vi "OPC UA Server.vi"() -> ()   [LabVIEW 2018]
uses:
  <vilib>/OPCUA/controls/Data Type.ctl
  <vilib>/OPCUA/NI OPC UA Server.lvlib
panel:
  in  "stop":bool
  out "Item Path":string
  out "Server Endpoint URL":string
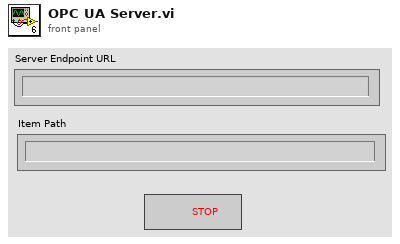
[diagram p1: front panel]
types:
  T1 = typedef "Data Type.ctl" = u16
  T2 = cluster{"name":string, "data type":T1, "access level":u16, "description":string}
  T3 = typedef "OPC UA Server Refnum.ctl" = refnum<k21>
  T4 = typedef "NodeId.ctl" = string
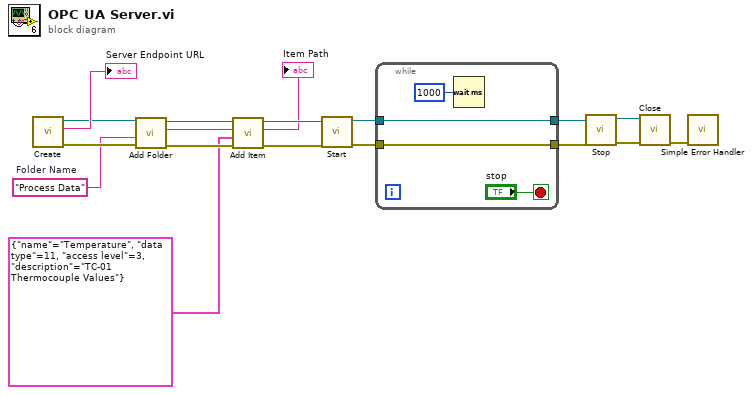
[diagram p0: block diagram]
diagram:
  w11 = "Process Data"  # Folder Name
  n1 = call <vilib>:"Create.vi"() -> ("error out"=w17:errorcluster, "server endpoint URL"=→"Server Endpoint URL":string, "OPC UA server refnum out"=w15:T3)  [unwired: 9 in]
  n2 = call <vilib>:"Add Folder.vi"("error in (no error)"=w17, "folder name"=w11, "OPC UA server refnum in"=w15) -> ("error out"=w16:errorcluster, "folder node ID"=w1:T4, "OPC UA server refnum out"=w14:T3)  [unwired: 5 in]
  n3 = call <vilib>:"Add Item.vi"("error in (no error)"=w16, "item"=T2 {"name"="Temperature", "data type"=11, "access level"=3, "description"="TC-01 Thermocouple Values"}, "parent folder node ID"=w1, "OPC UA server refnum in"=w14) -> ("error out"=w12:errorcluster, "item node ID"=→"Item Path":T4, "OPC UA server refnum out"=w13:T3)  [unwired: 3 in, 1 out]
  n4 = call <vilib>:"Start.vi"("error in (no error)"=w12, "OPC UA server refnum in"=w13) -> ("error out"=w8:errorcluster, "OPC UA server refnum out"=w6:T3)  [unwired: 7 in, 1 out]
  n5 = while {
    tunnel: w8 -> [w20]
    tunnel: [w20] -> w7
    tunnel: [w19] -> w5
    tunnel: w6 -> [w19]
    stop <- "stop" stop-if-true
    n6 = Wait (ms)(milliseconds to wait=u32 1000) -> ()  [unwired: 1 out]
  }
  n7 = call <vilib>:"Stop.vi"("error in (no error)"=w7, "OPC UA server refnum in"=w5) -> ("error out"=w4:errorcluster, "OPC UA server refnum out"=w3:T3)  [unwired: 8 in]
  n8 = call <vilib>:"Close.vi"("error in (no error)"=w4, "OPC UA server refnum in"=w3) -> ("error out"=w2:errorcluster)  [unwired: 9 in]
  n9 = call <vilib>:"Simple Error Handler.vi"("error in (no error)"=w2) -> ()  [unwired: 4 in, 5 out]
